vi "tablice_zadanie.vi"() -> ()   [LabVIEW 2012]
panel:
  out "Wartoœci I:":dbl[](array[numeric])
  out "i":dbl
  out "Wartoœci U:":dbl[](array[numeric])
  in  "Wartoœæ rezystancji":dbl
  # "Zbuduj program wyznaczaj¹cy Napiêcie  U  i Natê¿enie pr¹du I dla zadanego R \nzgodnie z prawem Ohma wyniki wyœwietl w tabeli  zawieraj¹cej U oraz I"
  # "Prgram wyznacza napiêcie i natê¿enie pr¹du dla zadanego R i losowych wartoœci natê¿enia lub napiêcia"
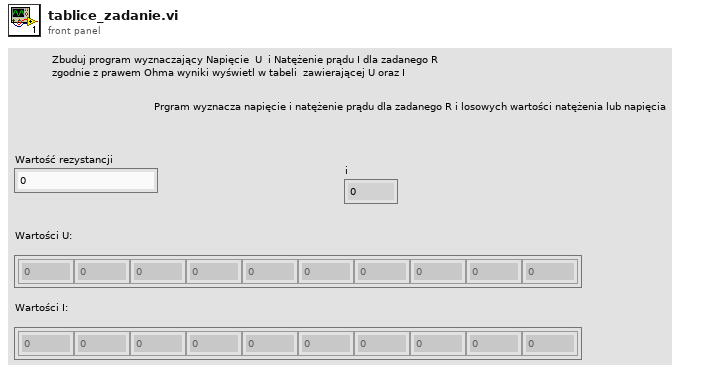
[diagram p1: front panel]
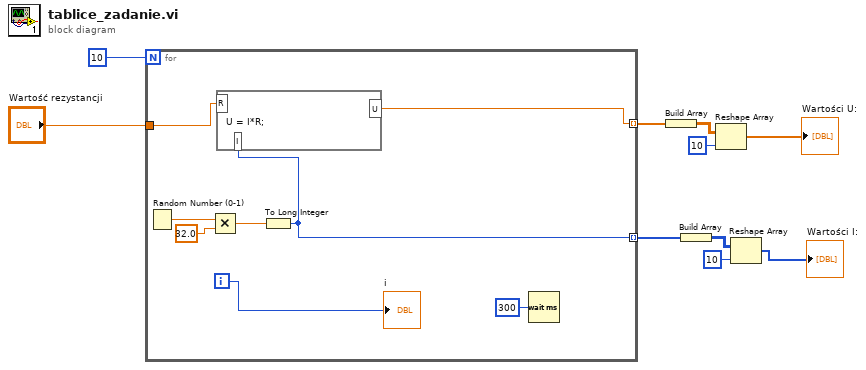
[diagram p0: block diagram]
diagram:
  n1 = for {
    N: 10 -> [_]
    tunnel: "Wartoœæ rezystancji" -> [w18]
    tunnel: [w15] -> w8 mode=indexing
    tunnel: [w11] -> w1 mode=indexing
    i -> [w16]
    n2 = Random Number (0-1)() -> (number: 0 to 1=w13:dbl)
    n3 = Multiply(x=w13, y=32.0) -> (x*y=w12:dbl)
    n4 = To Long Integer(number=w12) -> (32bit integer=w11:i32)
    n5 = formula code="U = I*R;"("I"=w11, "R"=w18) -> ("U"=w15:dbl)
    n6 = Wait (ms)(milliseconds to wait=u32 300) -> ()  [unwired: 1 out]
    "i" <- w16
  }
  n7 = Build Array(w8) -> (w7:dbl[][])
  n8 = Build Array(w1) -> (w4:i32[][])
  n9 = Reshape Array(w7, 10 ("dimension size")) -> (→"Wartoœci U:":dbl[])
  n10 = Reshape Array(w4, 10 ("dimension size")) -> (→"Wartoœci I:":i32[])
